vi "Actor Core.vi"(8 "error in":errorcluster, 11 "Simple UI in":refnum<class "Simple UI.lvclass">) -> (0 "error out":errorcluster, 3 "Actor out":refnum<class "Actor.lvclass">)   [LabVIEW 2020, in "Simple UI.lvlib" / "Simple UI.lvclass"]
doc: "<p>(<strong>Filename</strong>: <span class=\"dnl\">Actor Framework.lvlib:Actor.lvclass:Actor Core.vi</span>)</p>\n<p>Receives messages to the actor, reacts to them, and initiates any error handling that may shut the actor down.</p>\n<p>Descendant classes may override this VI to append parallel tasks for the actor to complete while it handles messages. Overrides use the <a href=\"nihelplauncher://docs/csh?context=lvcore_glang_udclass\">Call Parent Class Method</a> node.</p>"
uses:
  Simple UI.lvclass
  C:/Program Files/National Instruments/LabVIEW 2026/vi.lib/ActorFramework/Actor/Actor.lvclass
  <vilib>/ActorFramework/Actor/Actor.lvclass
  chart zoom.ctl
  Simple UI.lvclass/Simple UI.ctl
  <vilib>/ActorFramework/Actor/Actor.lvclass/Actor.ctl
  <vilib>/ActorFramework/Message Enqueuer/Message Enqueuer.lvclass/Message Enqueuer.ctl
  Application Manager/Application Manager Messages/Start Data Acquisition Msg/Start Data Acquisition Msg.lvclass/Start Data Acquisition Msg.ctl
  Application Manager/Application Manager Messages/Set CPU Calculation State Msg/Set CPU Calculation State Msg.lvclass/Set CPU Calculation State Msg.ctl
  Simple UI Messages/Write GPU View Msg/Write GPU View Msg.lvclass/Write GPU View Msg.ctl
  Simple UI Messages/Write CPU View Msg/Write CPU View Msg.lvclass/Write CPU View Msg.ctl
  Application Manager/Application Manager Messages/Set GPU FFT Config Msg/Set GPU FFT Config Msg.lvclass/Set GPU FFT Config Msg.ctl
  Application Manager/Application Manager Messages/Set GPU Calculation State Msg/Set GPU Calculation State Msg.lvclass/Set GPU Calculation State Msg.ctl
  Application Manager/Application Manager Messages/Set CPU FFT Config Msg/Set CPU FFT Config Msg.lvclass/Set CPU FFT Config Msg.ctl
  <vilib>/ActorFramework/Message Enqueuer/Enqueue.vi
  <vilib>/ActorFramework/Message Enqueuer/Init from Existing Queue.vi
  <vilib>/ActorFramework/Stop Msg/Stop Msg.lvclass
  C:/Program Files/National Instruments/LabVIEW 2026/vi.lib/ActorFramework/Message/Message.lvclass
  Application Manager/Application Manager Messages/Start Data Acquisition Msg/Start Data Acquisition Msg.lvclass
  Application Manager/Application Manager Messages/Set CPU Calculation State Msg/Set CPU Calculation State Msg.lvclass
  Simple UI Messages/Write GPU View Msg/Write GPU View Msg.lvclass
  Simple UI Messages/Write CPU View Msg/Write CPU View Msg.lvclass
  Application Manager/Application Manager Messages/Stop Data Acquisition Msg/Stop Data Acquisition Msg.lvclass
  Application Manager/Application Manager Messages/Start CPU Calculation Msg/Start CPU Calculation Msg.lvclass
  Application Manager/Application Manager Messages/Start GPU Calculation Msg/Start GPU Calculation Msg.lvclass
  Application Manager/Application Manager Messages/Set GPU FFT Config Msg/Set GPU FFT Config Msg.lvclass
  Application Manager/Application Manager Messages/Set GPU Calculation State Msg/Set GPU Calculation State Msg.lvclass
  Application Manager/Application Manager Messages/Set CPU FFT Config Msg/Set CPU FFT Config Msg.lvclass
  <vilib>/ActorFramework/Message Priority Queue/Priority Enqueue.vi
  Generic Actor/Generic Actor/Generic Actor.lvclass
  <vilib>/ActorFramework/Message Enqueuer/Message Enqueuer.lvclass
  <vilib>/ptbypt/NI_PtbyPt.lvlib
panel:
  out "Disk Read Datarate":waveform(dbl)(graph)
  in  "Continuous Disk":bool
  out "Data Source Info String":string
  out "FFT Rate Speedup":dbl caption="Elapsed Time:" format="FFT Rate Speedup %dx"
  out "Throughput Speedup":dbl caption="Elapsed Time:" format="Throughput Speedup %dx"
  in  "FFT Presets":T1(ring)
  out "CPU Equivalent FFT Time":waveform(dbl)(graph)
  out "GPU Equivalent FFT Time":waveform(dbl)(graph)
  in  "Load File":bool caption="Start Stop"
  out "GPU Throughput":waveform(dbl)(graph)
  in  "Continuous GPU":bool
  in  "Run GPU":bool caption="Start Stop"
  in  "Run CPU":bool caption="Start Stop"
  out "CPU Throughput":waveform(dbl)(graph)
  out "CPU to GPU Datarate":waveform(dbl)(graph)
  in  "Continuous CPU":bool
  out "GPU FFT Rate":dbl format="FFT Rate: %#_4pFFT/s"
  out "GPU Sampling Rate":dbl caption="Fs:" format="Fs: %#.3pHz"
  out "GPU Resolution Bandwidth":dbl caption="RBW:" format="RBW: %#.3pHz"
  out "GPU Done":bool caption="Done"
  out "GPU":dbl format="Throughput: %#_4dMS/s"
  out "GPU Elapsed Time":dbl caption="Elapsed Time:" format="Elapsed Time: %#.3gs"
  out "GPU Graph":cluster{dbl[], sgl[]}(graph)
  in  "GPU Batch Size":u64=100 min=1 max=1000 format="%.0p FFT"
  in  "GPU FFT Size":u64=2000000 min=128 format="%.0p Samples"
  in  "GPU View":T2 {"fwidth:" format="%#_6p"; "f0:" format="%#_6p"}
  out "CPU FFT Rate":dbl format="FFT Rate: %#_4pFFT/s"
  out "CPU Sampling Rate":dbl caption="Fs:" format="Fs: %#.3pHz"
  out "CPU Resolution Bandwidth":dbl caption="RBW:" format="RBW: %#.3pHz"
  out "CPU Done":bool caption="Done"
  out "CPU":dbl format="Throughput: %#_4dMS/s"
  out "CPU Elapsed Time":dbl caption="Elapsed Time:" format="Elapsed Time: %#.3gs"
  out "CPU Graph":cluster{dbl[], sgl[]}(graph)
  in  "CPU FFT Size":u64=2000000 min=128 format="%.0p Samples"
  in  "CPU View":T2 {"fwidth:" format="%#_6p"; "f0:" format="%#_6p"}
  # "Powered by"
  # "GPU FFT"
  # "GPU FFT"
  # "CPU FFT"
  # "CPU FFT"
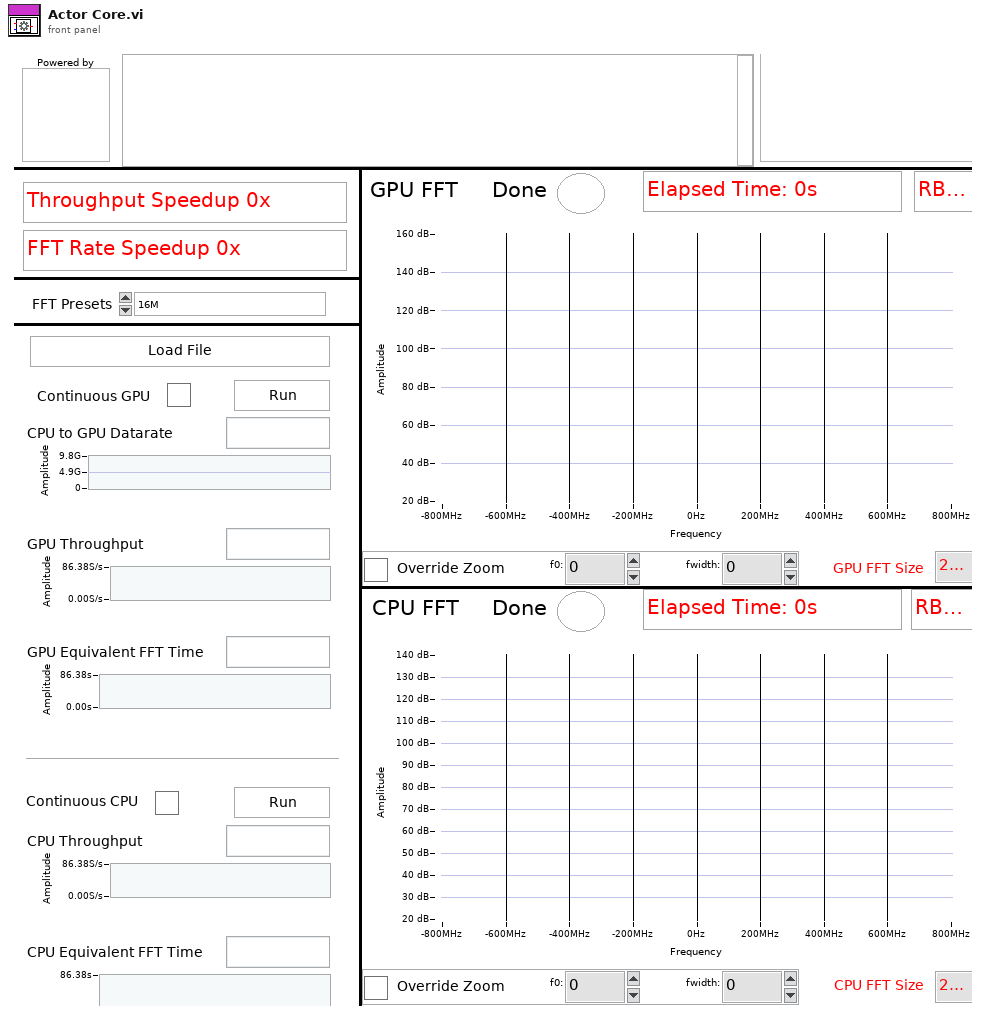
[diagram p1: front panel]
types:
  T1 = enum16{"16M", "4M", "2M", "1M", "512k", "128k", "4k", "2k", "1k"}
  T2 = typedef "Simple UI.lvlib/Simple UI.lvclass/chart zoom.ctl" = cluster{"Override":bool, "f0: ":dbl, "fwidth: ":dbl}
  T3 = enum32{"Invalid", "Standard", "Closed", "Hidden", "Minimized", "Maximized"}
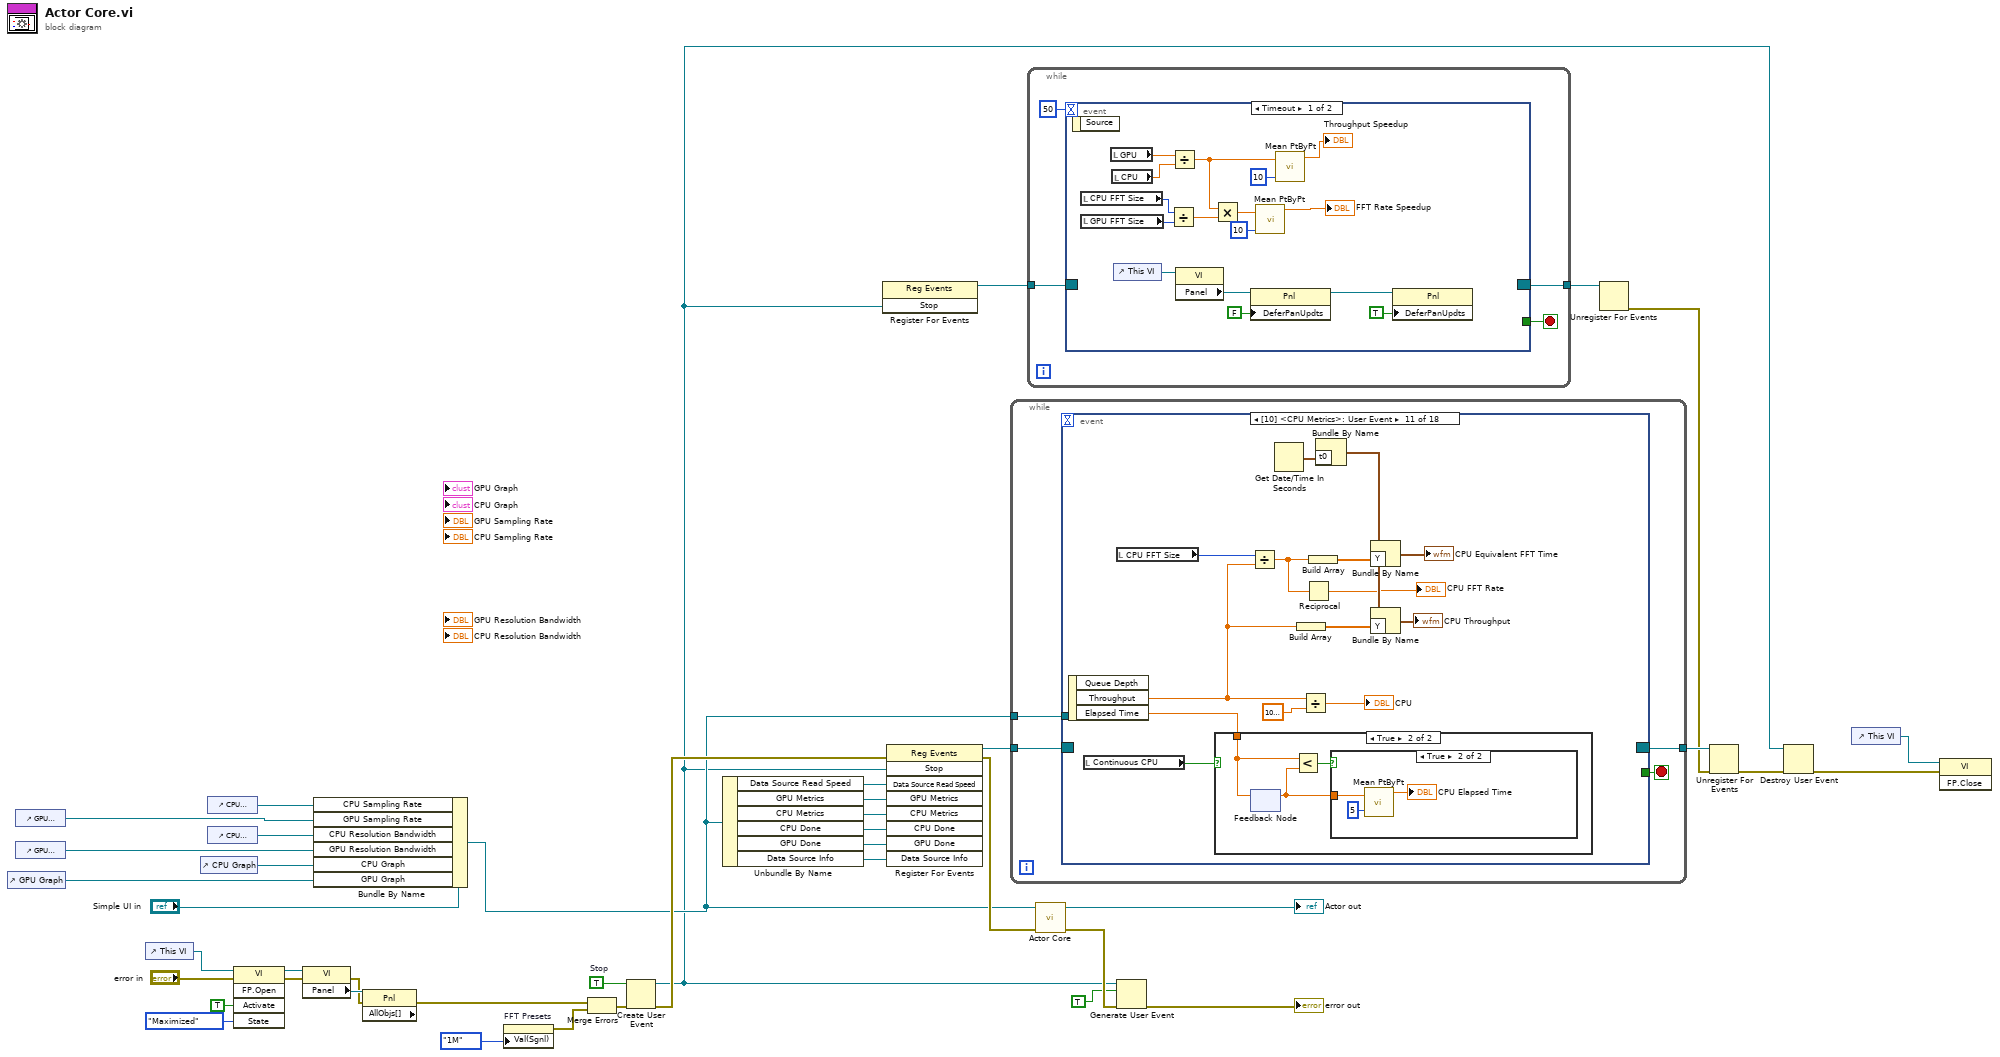
[diagram p0: block diagram]
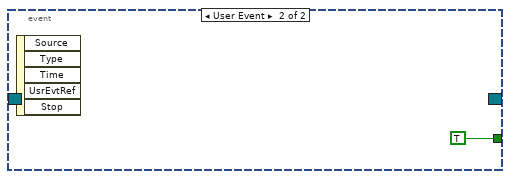
[diagram p2: hidden frame]
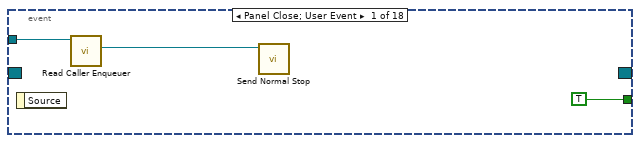
[diagram p3: hidden frame]
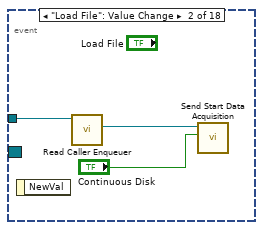
[diagram p4: hidden frame]
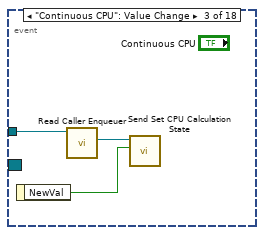
[diagram p5: hidden frame]
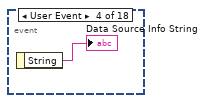
[diagram p6: hidden frame]
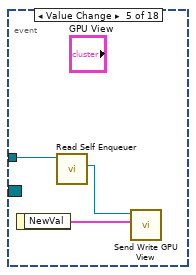
[diagram p7: hidden frame]
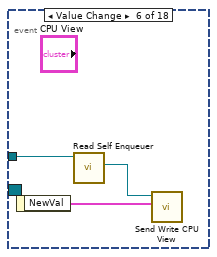
[diagram p8: hidden frame]
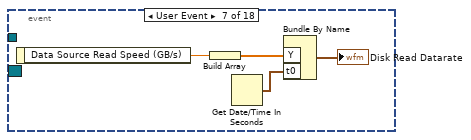
[diagram p9: hidden frame]
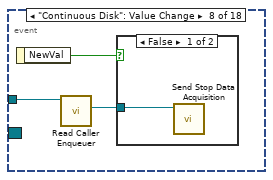
[diagram p10: hidden frame]
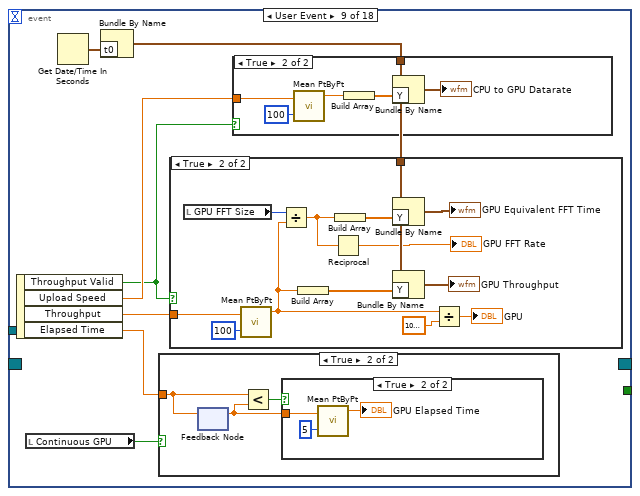
[diagram p12: hidden frame]
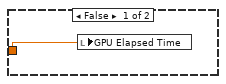
[diagram p15: hidden frame]
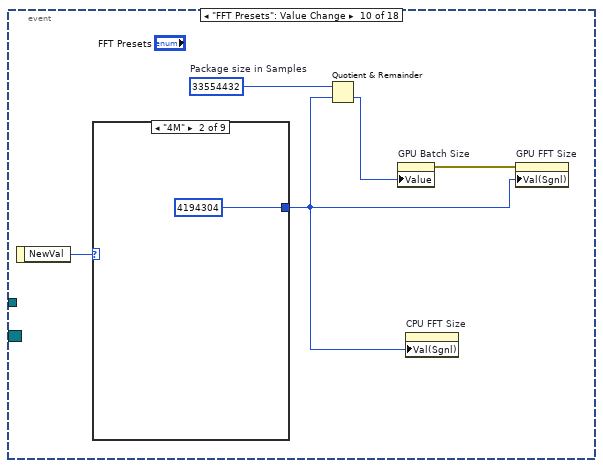
[diagram p17: hidden frame]
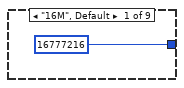
[diagram p18: hidden frame]
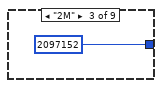
[diagram p19: hidden frame]
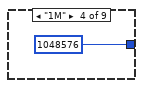
[diagram p20: hidden frame]
diagram:
  w42 = TRUE  # Stop
  n1 = control-ref of="GPU Graph"() -> (w29:refnum<vi>)
  n2 = control-ref of="GPU Sampling Rate"() -> (w21:refnum<vi>)
  n3 = control-ref of="GPU Resolution Bandwidth"() -> (w24:refnum<vi>)
  n4 = control-ref of="This VI"() -> (w12:refnum<vi>)
  n5 = control-ref of="CPU Graph"() -> (w30:refnum<vi>)
  n6 = control-ref of="CPU Sampling Rate"() -> (w22:refnum<vi>)
  n7 = control-ref of="CPU Resolution Bandwidth"() -> (w23:refnum<vi>)
  n8 = invoke class="VI" method="FP.Open"(reference=w12, error in="error in", "Activate"=TRUE ("Activate?"), "State"=T3."Maximized") -> (reference out=w7:refnum<vi>, error out=w5:errorcluster)  [unwired: 1 in, 3 out]
  n9 = property class="VI"(reference=w7, error in=w5) -> (error out=w4:errorcluster, "Panel"=w6:refnum<vi>)  [unwired: 1 out]
  n10 = Bundle By Name(cluster="Simple UI in", "CPU Sampling Rate"=w22, "GPU Sampling Rate"=w21, "CPU Resolution Bandwidth"=w23, "GPU Resolution Bandwidth"=w24, "CPU Graph"=w30, "GPU Graph"=w29) -> (w31:refnum<class "Simple UI.lvclass">)
  n11 = property class="Pnl" props=["AllObjs[]"](reference=w6, error in=w4) -> (error out=w1:errorcluster)  [unwired: 2 out]
  n12 = property on="FFT Presets" class="Enum (strict)"("Val(Sgnl)"=T1."1M" ("FFT Presets")) -> (error out=w3:errorcluster)  [unwired: 2 in, 1 out]
  n13 = Merge Errors(w1, w3) -> (w17:errorcluster)
  n14 = Create User Event(user event datatype=w42, error in=w17) -> (user event=w27:refnum<user-event>, error out=w41:errorcluster)
  n15 = Unbundle By Name(w31) -> ("Data Source Read Speed"=w34:refnum<user-event>, "GPU Metrics"=w33:refnum<user-event>, "CPU Metrics"=w32:refnum<user-event>, "CPU Done"=w20:refnum<user-event>, "GPU Done"=w19:refnum<user-event>, "Data Source Info"=w18:refnum<user-event>)
  n16 = register-events(w27) -> (reference out=w26:refnum<event-registration>)  [unwired: 2 in, 1 out]
  n17 = register-events(error in=w41, w27, w34, w33, w32, w20, w19, w18) -> (reference out=w40:refnum<event-registration>, error out=w38:errorcluster)  [unwired: 1 in]
  n18 = while {
    tunnel: w31 -> [w45]
    tunnel: w40 -> [w44]
    tunnel: [w43] -> w39
    stop <- w46 stop-if-true
    n19 = event shown="[10] <CPU Metrics>: User Event" {
      selector: w44 -> [_ _ _ _ _ _ _ _ _ _ _ _ _ _ _ _ _ _]
      dyn-events: [_ _ _ _ _ _ _ _ _ _ _ _ _ _ _ _ _ _] -> w43
      timeout: _ -> [_ _ _ _ _ _ _ _ _ _ _ _ _ _ _ _ _ _]
      tunnel: [TRUE _ _ _ _ _ _ _ _ _ _ _ _ _ _ _ _ _] -> w46
      tunnel: w45 -> [w48 w52 w55 _ w58 w62 _ w68 _ _ _ w140 w142 w144 w149 w152 _ _]
      event Panel Close; User Event {
        n20 = event-data() -> ()  [unwired: 1 in, 1 out]
        n21 = call <vilib>:"Read Caller Enqueuer.vi"("Actor"=w48) -> ("Caller Enqueuer"=w47:refnum<class "Message Enqueuer.lvclass">)  [unwired: 10 in]
        n22 = call <vilib>:"Send Normal Stop.vi"("Message Enqueuer"=w47) -> ()  [unwired: 10 in, 1 out]
      }
      event "Load File": Value Change {
        n23 = event-data() -> ()  [unwired: 1 in, 1 out]
        n24 = call <vilib>:"Read Caller Enqueuer.vi"("Actor"=w52) -> ("Caller Enqueuer"=w51:refnum<class "Message Enqueuer.lvclass">)  [unwired: 10 in]
        n25 = call "Send Start Data Acquisition.vi"("Continuous"="Continuous Disk", "Message Enqueuer"=w51) -> ()  [unwired: 8 in, 2 out]
      }
      event "Continuous CPU": Value Change {
        n26 = event-data() -> ("NewVal"=w53:bool)  [unwired: 1 in]
        n27 = call <vilib>:"Read Caller Enqueuer.vi"("Actor"=w55) -> ("Caller Enqueuer"=w54:refnum<class "Message Enqueuer.lvclass">)  [unwired: 10 in]
        n28 = call "Send Set CPU Calculation State.vi"("Continuous"=w53, "Message Enqueuer"=w54) -> ()  [unwired: 8 in, 2 out]
      }
      event User Event {
        n29 = event-data() -> ("String"=→"Data Source Info String":string)  [unwired: 1 in]
      }
      event Value Change {
        n30 = event-data() -> ("NewVal"=w59:T2)  [unwired: 1 in]
        n31 = call <vilib>:"Read Self Enqueuer.vi"("Actor"=w58) -> ("Self Enqueuer"=w57:refnum<class "Message Enqueuer.lvclass">)  [unwired: 10 in]
        n32 = call "Send Write GPU View.vi"("CPU View"=w59, "Message Enqueuer"=w57) -> ()  [unwired: 8 in, 2 out]
      }
      event Value Change {
        n33 = event-data() -> ("NewVal"=w60:T2)  [unwired: 1 in]
        n34 = call <vilib>:"Read Self Enqueuer.vi"("Actor"=w62) -> ("Self Enqueuer"=w61:refnum<class "Message Enqueuer.lvclass">)  [unwired: 10 in]
        n35 = call "Send Write CPU View.vi"("CPU View"=w60, "Message Enqueuer"=w61) -> ()  [unwired: 8 in, 2 out]
      }
      event User Event {
        n36 = event-data() -> ("Data Source Read Speed (GB/s)"=w66:dbl)  [unwired: 1 in]
        n37 = Build Array(w66) -> (w64:dbl[])
        n38 = Get Date/Time In Seconds() -> (seconds since 1Jan1904=w63:timestamp)
        n39 = Bundle By Name("Y"=w64, "t0"=w63) -> (→"Disk Read Datarate":waveform(dbl))  [unwired: 1 in]
      }
      event "Continuous Disk": Value Change {
        n40 = event-data() -> ("NewVal"=w69:bool)  [unwired: 1 in]
        n41 = call <vilib>:"Read Caller Enqueuer.vi"("Actor"=w68) -> ("Caller Enqueuer"=w67:refnum<class "Message Enqueuer.lvclass">)  [unwired: 10 in]
        n42 = case shown="False" w69 {
          tunnel: w67 -> [w70 _]
          frame False {
            n43 = call "Send Stop Data Acquisition.vi"("Message Enqueuer"=w70) -> ()  [unwired: 9 in, 2 out]
          }
          frame True {
          }
        }
      }
      event User Event {
        n44 = event-data() -> ("Throughput Valid"=w71:bool, "Upload Speed"=w72:dbl, "Throughput"=w74:dbl, "Elapsed Time"=w76:dbl)  [unwired: 1 in]
        n45 = local read "Continuous GPU"() -> (w75:bool)
        n46 = Get Date/Time In Seconds() -> (seconds since 1Jan1904=w77:timestamp)
        n47 = Bundle By Name("t0"=w77) -> (w73:waveform(dbl))  [unwired: 1 in]
        n48 = case shown="True" w75 {
          tunnel: w76 -> [w97 w100]
          frame False {
            n49 = local write "GPU Elapsed Time"(w97) -> ()
          }
          frame True {
            n50 = feedback #1() -> (w98:dbl)  [unwired: 1 in]
            n51 = feedback-in #1(w100) -> ()
            n52 = Less?(x=w100, y=w98) -> (x < y?=w99:bool)
            n53 = case shown="True" w99 {
              tunnel: w98 -> [_ w103]
              frame False {
              }
              frame True {
                n54 = call <vilib>:"Mean PtByPt.vi"("x"=w103, "sample length"=5) -> ("mean"=→"GPU Elapsed Time":dbl)  [unwired: 2 in, 1 out]
              }
            }
          }
        }
        n55 = case shown="True" w71 {
          tunnel: w74 -> [_ w92]
          tunnel: w73 -> [_ w91]
          frame False {
          }
          frame True {
            n56 = local read "GPU FFT Size"() -> (w89:u64)
            n57 = call <vilib>:"Mean PtByPt.vi"("x"=w92, "sample length"=100) -> ("mean"=w87:dbl)  [unwired: 2 in, 1 out]
            n58 = Divide(x=w89, y=w87) -> (x/y=w85:dbl)
            n59 = Build Array(w87) -> (w88:dbl[])
            n60 = Reciprocal(x=w85) -> (1/x=→"GPU FFT Rate":dbl)
            n61 = Build Array(w85) -> (w86:dbl[])
            n62 = Bundle By Name(cluster=w91, "Y"=w86) -> (→"GPU Equivalent FFT Time":waveform(dbl))
            n63 = Bundle By Name(cluster=w91, "Y"=w88) -> (→"GPU Throughput":waveform(dbl))
            n64 = Divide(x=w87, y=1000000.0 ("x")) -> (x/y=→"GPU":dbl)
          }
        }
        n65 = case shown="True" w71 {
          tunnel: w73 -> [_ w82]
          tunnel: w72 -> [_ w78]
          frame False {
          }
          frame True {
            n66 = call <vilib>:"Mean PtByPt.vi"("x"=w78, "sample length"=100) -> ("mean"=w80:dbl)  [unwired: 2 in, 1 out]
            n67 = Build Array(w80) -> (w79:dbl[])
            n68 = Bundle By Name(cluster=w82, "Y"=w79) -> (→"CPU to GPU Datarate":waveform(dbl))
          }
        }
      }
      event "FFT Presets": Value Change {
        w106 = u64 33554432  # Package size in Samples
        n69 = event-data() -> ("NewVal"=w108:T1)  [unwired: 1 in]
        n70 = case shown="\"4M\"" w108 {
          tunnel: [u64 16777216 u64 4194304 u64 2097152 u64 1048576 u64 524288 u64 131072 u64 4096 u64 2048 u64 1024] -> w105
          frame "16M", Default {
          }
          frame "4M" {
          }
          frame "2M" {
          }
          frame "1M" {
          }
          frame "512k" {
          }
          frame "128k" {
          }
          frame "4k" {
          }
          frame "2k" {
          }
          frame "1k" {
          }
        }
        n71 = Quotient & Remainder(x=w106, y=w105) -> (floor(x/y)=w104:u64)  [unwired: 1 out]
        n72 = property on="GPU Batch Size" class="DigNum (strict)"("Value"=w104) -> (error out=w107:errorcluster)  [unwired: 2 in, 1 out]
        n73 = property on="CPU FFT Size" class="DigNum (strict)"("Val(Sgnl)"=w105) -> ()  [unwired: 2 in, 2 out]
        n74 = property on="GPU FFT Size" class="DigNum (strict)"(error in=w107, "Val(Sgnl)"=w105) -> ()  [unwired: 1 in, 2 out]
      }
      event User Event {
        n75 = event-data() -> ("Throughput"=w125:dbl, "Elapsed Time"=w127:dbl)  [unwired: 1 in, 1 out]
        n76 = local read "Continuous CPU"() -> (w126:bool)
        n77 = local read "CPU FFT Size"() -> (w122:u64)
        n78 = case shown="True" w126 {
          tunnel: w127 -> [w132 w135]
          frame False {
            n79 = local write "CPU Elapsed Time"(w132) -> ()
          }
          frame True {
            n80 = feedback #2() -> (w133:dbl)  [unwired: 1 in]
            n81 = feedback-in #2(w135) -> ()
            n82 = Less?(x=w135, y=w133) -> (x < y?=w134:bool)
            n83 = case shown="True" w134 {
              tunnel: w133 -> [_ w138]
              frame False {
              }
              frame True {
                n84 = call <vilib>:"Mean PtByPt.vi"("x"=w138, "sample length"=5) -> ("mean"=→"CPU Elapsed Time":dbl)  [unwired: 2 in, 1 out]
              }
            }
          }
        }
        n85 = Divide(x=w122, y=w125) -> (x/y=w119:dbl)
        n86 = Get Date/Time In Seconds() -> (seconds since 1Jan1904=w131:timestamp)
        n87 = Build Array(w125) -> (w121:dbl[])
        n88 = Divide(x=w125, y=1000000.0 ("x")) -> (x/y=→"CPU":dbl)
        n89 = Reciprocal(x=w119) -> (1/x=→"CPU FFT Rate":dbl)
        n90 = Build Array(w119) -> (w120:dbl[])
        n91 = Bundle By Name("t0"=w131) -> (w124:waveform(dbl))  [unwired: 1 in]
        n92 = Bundle By Name(cluster=w124, "Y"=w120) -> (→"CPU Equivalent FFT Time":waveform(dbl))
        n93 = Bundle By Name(cluster=w124, "Y"=w121) -> (→"CPU Throughput":waveform(dbl))
      }
      event "Run CPU": Value Change {
        n94 = event-data() -> ()  [unwired: 1 in, 1 out]
        n95 = call <vilib>:"Read Caller Enqueuer.vi"("Actor"=w140) -> ("Caller Enqueuer"=w139:refnum<class "Message Enqueuer.lvclass">)  [unwired: 10 in]
        n96 = call "Send Start CPU Calculation.vi"("Message Enqueuer"=w139) -> ()  [unwired: 9 in, 2 out]
      }
      event "Run GPU": Value Change {
        n97 = event-data() -> ()  [unwired: 1 in, 1 out]
        n98 = call <vilib>:"Read Caller Enqueuer.vi"("Actor"=w142) -> ("Caller Enqueuer"=w141:refnum<class "Message Enqueuer.lvclass">)  [unwired: 10 in]
        n99 = call "Send Start GPU Calculation.vi"("Message Enqueuer"=w141) -> ()  [unwired: 9 in, 2 out]
      }
      event "GPU FFT Size", "GPU Batch Size": Value Change {
        n100 = event-data() -> ()  [unwired: 1 in, 4 out]
        n101 = call <vilib>:"Read Caller Enqueuer.vi"("Actor"=w144) -> ("Caller Enqueuer"=w143:refnum<class "Message Enqueuer.lvclass">)  [unwired: 10 in]
        n102 = call "Send Set GPU FFT Config.vi"("Batch Size"="GPU Batch Size", "FFT Size"="GPU FFT Size", "Message Enqueuer"=w143) -> ()  [unwired: 7 in, 2 out]
      }
      event "Continuous GPU": Value Change {
        n103 = event-data() -> ("NewVal"=w147:bool)  [unwired: 1 in]
        n104 = call <vilib>:"Read Caller Enqueuer.vi"("Actor"=w149) -> ("Caller Enqueuer"=w148:refnum<class "Message Enqueuer.lvclass">)  [unwired: 10 in]
        n105 = call "Send Set GPU Calculation State.vi"("Continuous"=w147, "Message Enqueuer"=w148) -> ()  [unwired: 8 in, 2 out]
      }
      event "CPU FFT Size": Value Change {
        n106 = event-data() -> ()  [unwired: 1 in, 4 out]
        n107 = call <vilib>:"Read Caller Enqueuer.vi"("Actor"=w152) -> ("Caller Enqueuer"=w151:refnum<class "Message Enqueuer.lvclass">)  [unwired: 10 in]
        n108 = call "Send Set CPU FFT Config.vi"("CPU FFT Size"="CPU FFT Size", "Message Enqueuer"=w151) -> ()  [unwired: 8 in, 2 out]
      }
      event User Event {
        n109 = event-data() -> ("CPU Done"=→"CPU Done":bool)  [unwired: 1 in]
      }
      event User Event {
        n110 = event-data() -> ("GPU Done"=→"GPU Done":bool)  [unwired: 1 in]
      }
    }
  }
  n111 = while {
    tunnel: [w157] -> w28
    tunnel: w26 -> [w158]
    stop <- w156 stop-if-true
    n112 = event shown="[0] Timeout" {
      selector: w158 -> [_ _]
      dyn-events: [_ _] -> w157
      timeout: 50 -> [_ _]
      tunnel: [_ TRUE] -> w156
      event Timeout {
        n113 = event-data() -> ()  [unwired: 1 in, 1 out]
        n114 = local read "CPU FFT Size"() -> (w163:u64)
        n115 = local read "GPU FFT Size"() -> (w164:u64)
        n116 = local read "GPU"() -> (w169:dbl)
        n117 = local read "CPU"() -> (w168:dbl)
        n118 = control-ref of="This VI"() -> (w174:refnum<vi>)
        n119 = Divide(x=w163, y=w164) -> (x/y=w162:dbl)
        n120 = Divide(x=w169, y=w168) -> (x/y=w161:dbl)
        n121 = property class="VI"(reference=w174) -> ("Panel"=w173:refnum<vi>)  [unwired: 1 in, 2 out]
        n122 = Multiply(x=w161, y=w162) -> (x*y=w160:dbl)
        n123 = property class="Pnl"(reference=w173, "DeferPanUpdts"=FALSE ("Defer Panel Updates")) -> (reference out=w171:refnum<vi>)  [unwired: 1 in, 1 out]
        n124 = call <vilib>:"Mean PtByPt.vi"("x"=w160, "sample length"=10) -> ("mean"=→"FFT Rate Speedup":dbl)  [unwired: 2 in, 1 out]
        n125 = call <vilib>:"Mean PtByPt.vi"("x"=w161, "sample length"=10) -> ("mean"=→"Throughput Speedup":dbl)  [unwired: 2 in, 1 out]
        n126 = property class="Pnl"(reference=w171, "DeferPanUpdts"=TRUE ("Defer Panel Updates")) -> ()  [unwired: 1 in, 2 out]
      }
      event User Event {
        n127 = event-data() -> ()  [unwired: 1 in, 5 out]
      }
    }
  }
  n128 = call-parent "Actor Core.vi"("error in"=w38, "Actor in"=w31) -> ("error out"=w36:errorcluster, "Actor out"=→"Actor out":refnum<class "Actor.lvclass">)  [unwired: 8 in]
  n129 = Generate User Event(user event=w27, event data cluster=TRUE ("event data"), error in=w36) -> (error out=→"error out":errorcluster)  [unwired: 1 in, 1 out]
  n130 = Unregister For Events(event registration refnum=w28) -> (error out=w25:errorcluster)  [unwired: 1 in]
  n131 = Unregister For Events(event registration refnum=w39, error in=w25) -> (error out=w37:errorcluster)
  n132 = Destroy User Event(user event=w27, error in=w37) -> (error out=w10:errorcluster)
  n133 = control-ref of="This VI"() -> (w11:refnum<vi>)
  n134 = invoke class="VI" method="FP.Close"(reference=w11, error in=w10) -> ()  [unwired: 1 in, 3 out]
